vi "TurboValve_control.vi"(6 "Bool Refnum":refnum<vi>, 7 "Spec turbo\nvalve ctrl":bool, 9 "FieldPoint IO Point":refnum<k21>, 10 "FieldPoint IO Point 2":refnum<k21>, 11 "Boolean in":refnum<vi>) -> (0 "error out":errorcluster, 1 "Spec Open":errorcluster caption="error out", 2 "Spec Close":errorcluster caption="error out", 3 "Boolean 9":bool, 5 "Boolean 8":bool)   [LabVIEW 2014]
uses:
  <vilib>/FieldPoint/Polymorphic Write.llb/FP Write (Boolean -IO).vi
  <vilib>/FieldPoint/Polymorphic Read.llb/FP Read (Boolean -IO).vi
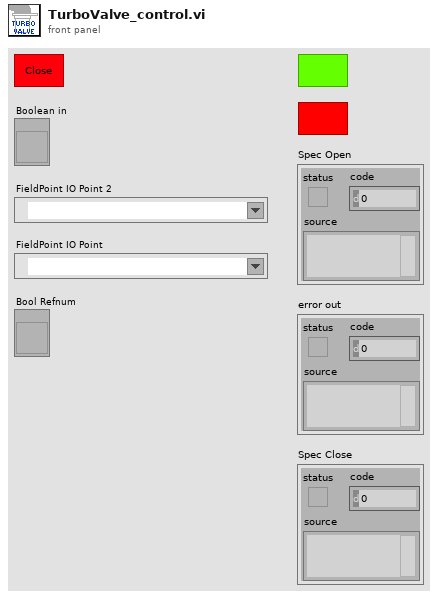
[diagram p1: front panel]
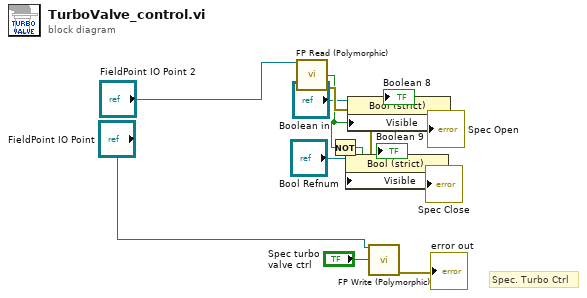
[diagram p0: block diagram]
diagram:
  # "Spec. Turbo Ctrl"
  n1 = call-poly <vilib>:"FP Read (Polymorphic).vi"("FieldPoint IO Point In"="FieldPoint IO Point 2") -> ("value"=w3:bool, "error out"=w6:errorcluster)  [unwired: 11 in, 2 out]
  n2 = Not(x=w3) -> (.not. x?=w4:bool)
  n3 = property on="Property Node" class="Bool (strict)"(reference="Bool Refnum", error in=w6, "Visible"=w4) -> (error out=→"Spec Close":errorcluster)  [unwired: 1 out]
  n4 = property on="Property Node" class="Bool (strict)"(reference="Boolean in", error in=w6, "Visible"=w3) -> (error out=→"Spec Open":errorcluster)  [unwired: 1 out]
  n5 = call-poly <vilib>:"FP Write (Polymorphic).vi"("FieldPoint IO Point In"="FieldPoint IO Point", "value"="Spec turbo\nvalve ctrl") -> ("error out"=→"error out":errorcluster)  [unwired: 11 in, 2 out]
